vi "InitConfig.vi"() -> ()   [LabVIEW 2014]
uses:
  QMH Fundamentals - Message Cluster.ctl
panel:
  in  "返回2":bool
  in  "标准测试":bool
  in  "自定义测试":bool
  in  "返回":bool
  in  "自动测试":bool
  in  "单次测试":bool
  in  "自定义测试":bool
  in  "常温拷机":bool
  in  "高温老练":bool
  in  "温循":bool
  in  "退出":bool
  in  "手动测试":bool
  in  "全自动测试":bool
  # "请选择测试类型"
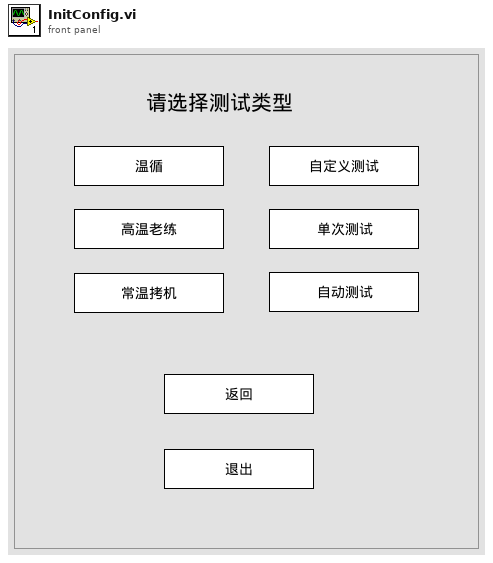
[diagram p1: front panel]
types:
  T1 = typedef "QMH Fundamentals - Message Cluster.ctl" = cluster{"消息":string, "消息数据":variant}
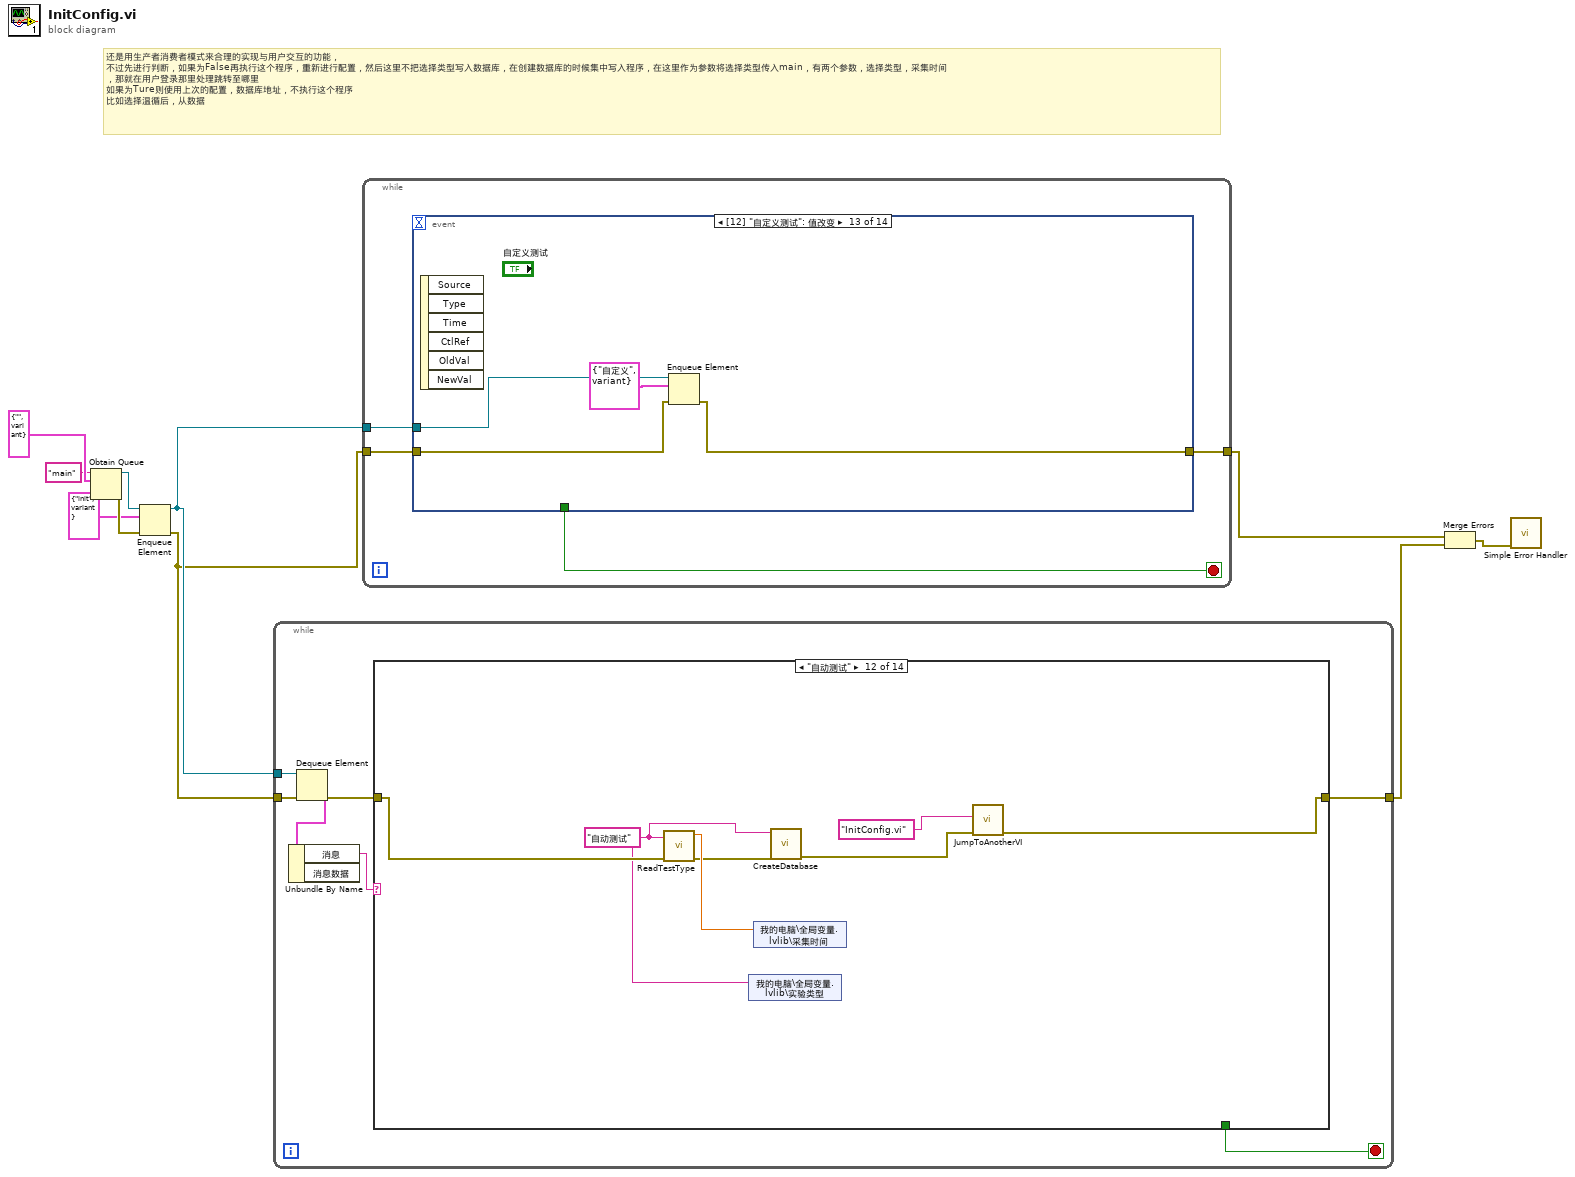
[diagram p0: block diagram]
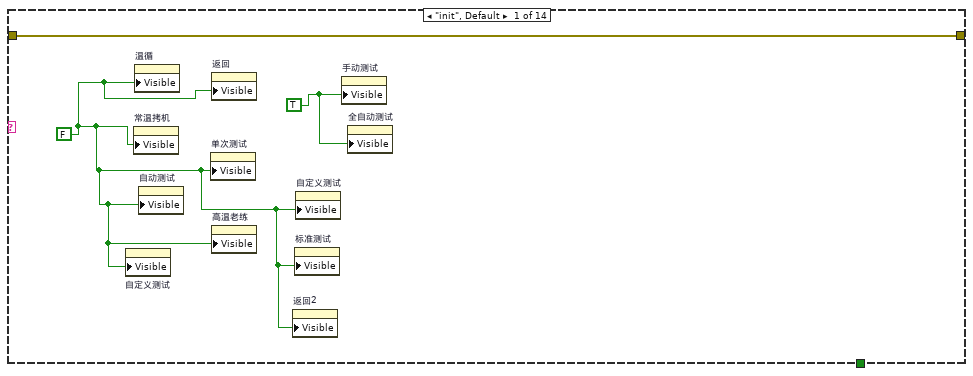
[diagram p2: hidden frame]
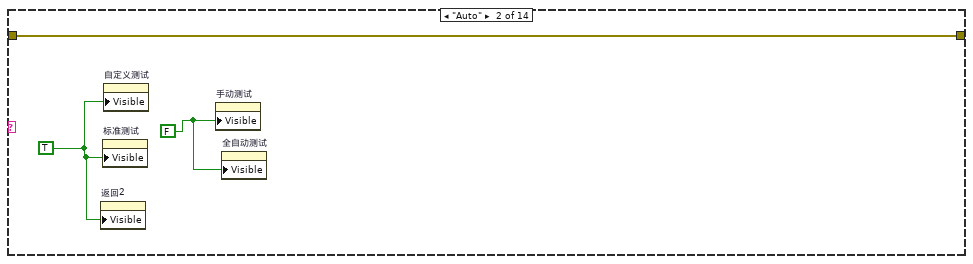
[diagram p3: hidden frame]
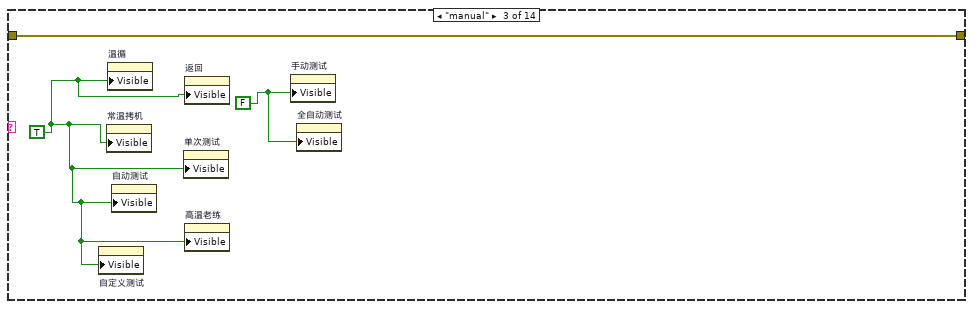
[diagram p4: hidden frame]
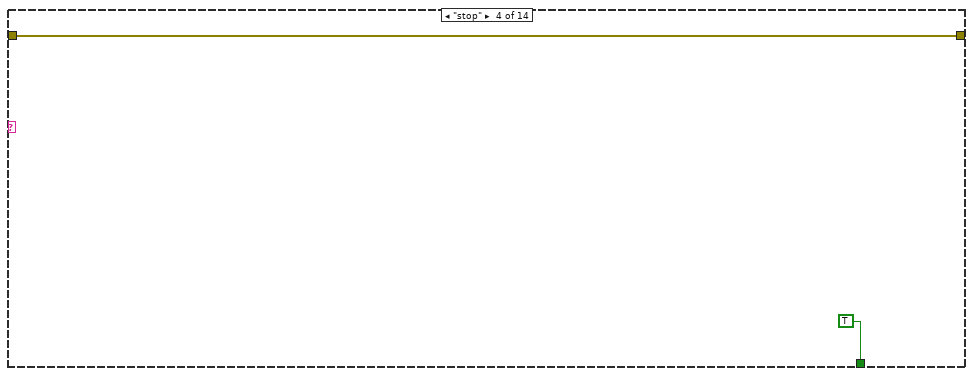
[diagram p5: hidden frame]
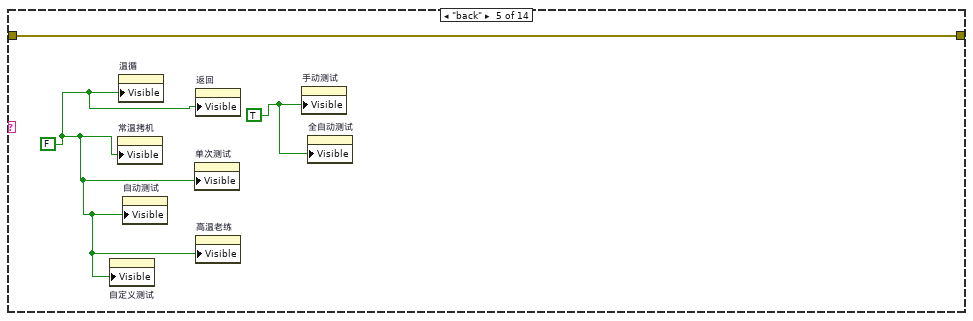
[diagram p6: hidden frame]
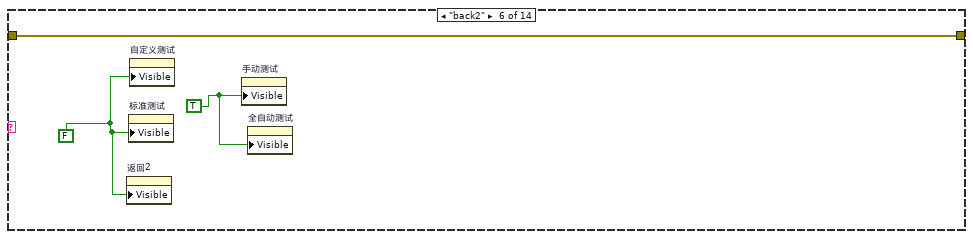
[diagram p7: hidden frame]
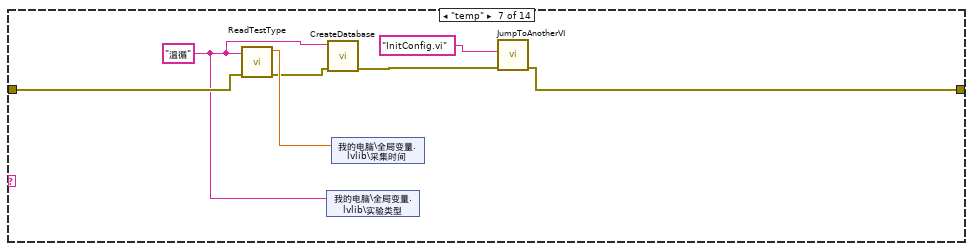
[diagram p8: hidden frame]
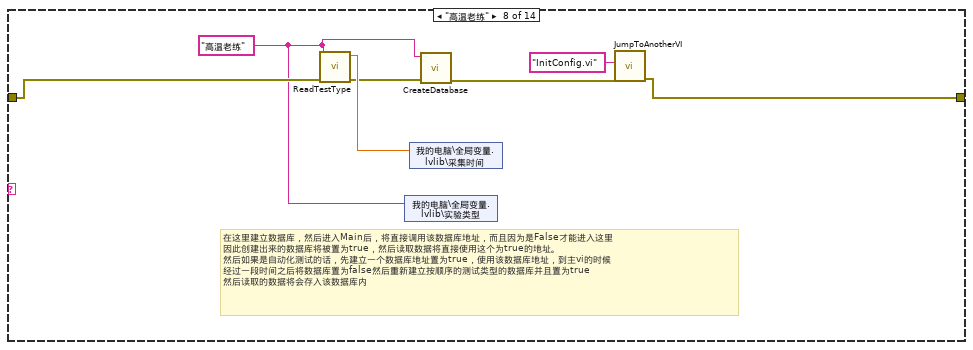
[diagram p9: hidden frame]
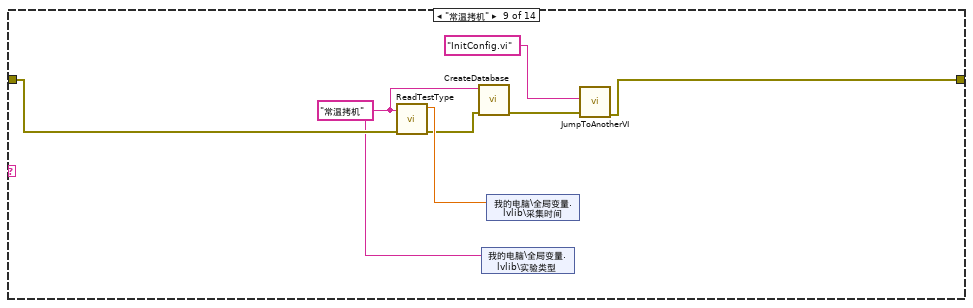
[diagram p10: hidden frame]
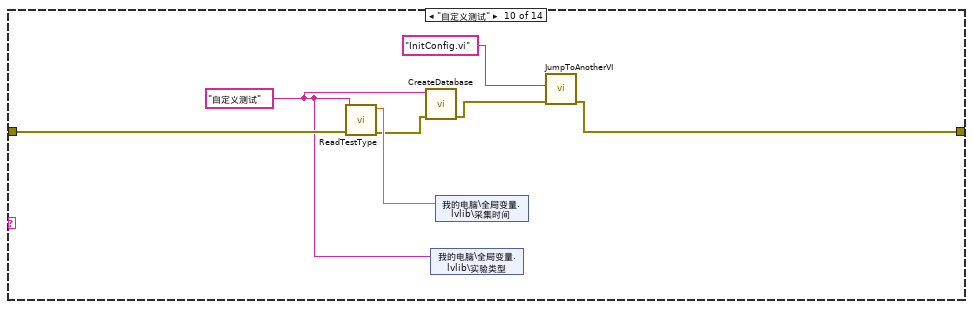
[diagram p11: hidden frame]
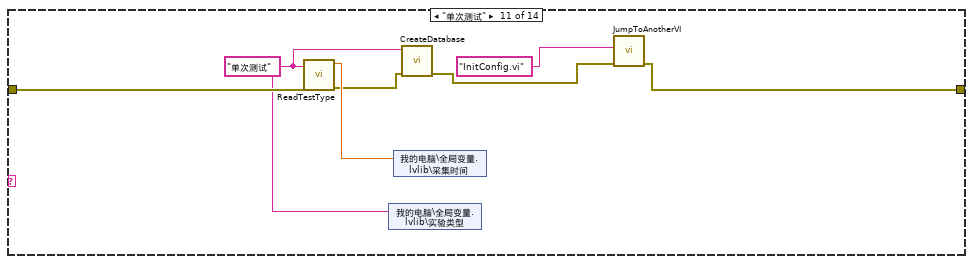
[diagram p12: hidden frame]
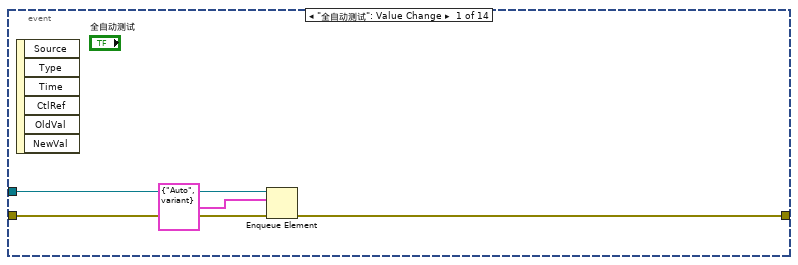
[diagram p15: hidden frame]
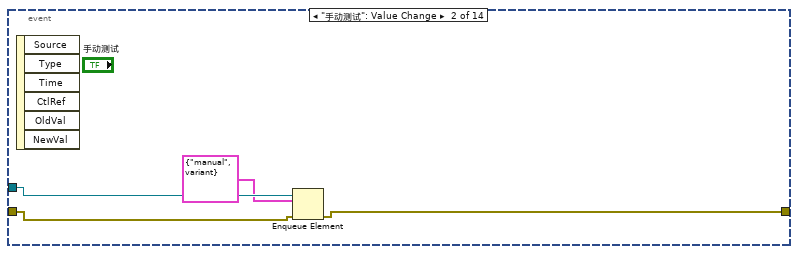
[diagram p16: hidden frame]
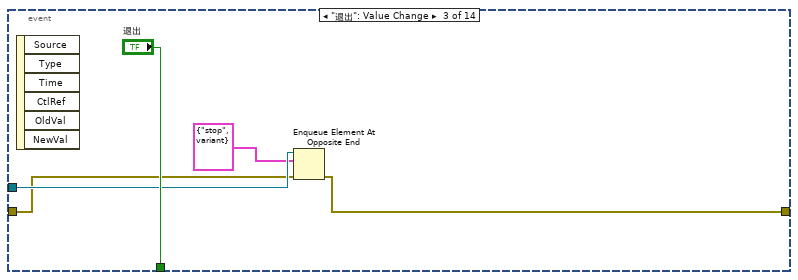
[diagram p17: hidden frame]
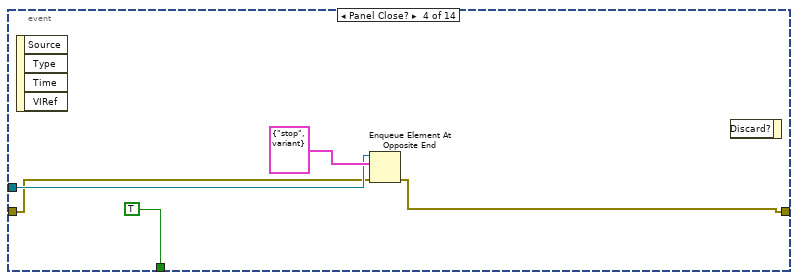
[diagram p18: hidden frame]
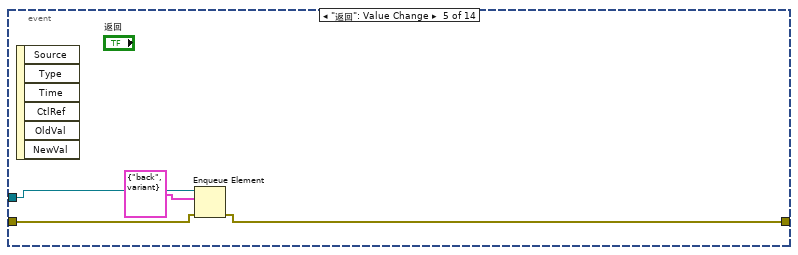
[diagram p19: hidden frame]
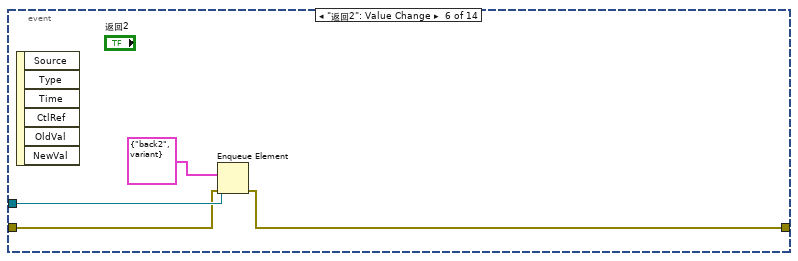
[diagram p20: hidden frame]
diagram:
  # "还是用生产者消费者模式来合理的实现与用户交互的功能，\n不过先进行判断，如果为False再执行这个程序，重新进行配置，然后这里不把选择类型写入数据库，在创建数据库的时候集中写入程序，在这里作为参数将选择类型传入main，有两个参数，选择类型，采集时间\n，那就在用户登录那里处理跳转至哪里\n如果为Ture则使用上次的配置，数据库地址，不执行这个程序\n比如选择温循后，从数据"
  n1 = Obtain Queue(name (unnamed)="main" ("名称（未命名）"), element data type=T1 {"消息"="", "消息数据"=variant} ("消息簇")) -> (queue out=w8:refnum<queue>, error out=w7:errorcluster)  [unwired: 3 in, 1 out]
  n2 = Enqueue Element(queue=w8, element=T1 {"消息"="init", "消息数据"=variant} ("元素"), error in (no error)=w7) -> (queue out=w5:refnum<queue>, error out=w4:errorcluster)  [unwired: 1 in, 1 out]
  n3 = while {
    tunnel: w5 -> [w17]
    tunnel: w4 -> [w16]
    tunnel: [w12] -> w2
    stop <- w11 stop-if-true
    n4 = Dequeue Element(queue=w17, error in (no error)=w16) -> (element=w15:T1, error out=w13:errorcluster)  [unwired: 1 in, 2 out]
    n5 = Unbundle By Name(w15) -> ("消息"=w14:string)  [unwired: 1 out]
    n6 = case shown="\"自动测试\"" w14 {
      tunnel: w13 -> [w20 w23 w26 w28 w29 w32 w41 w47 w54 w61 w68 w75 w77 w78]
      tunnel: [w20 w23 w26 w28 w29 w32 w39 w46 w53 w60 w67 w74 w77 w78] -> w12
      tunnel: [_ _ _ TRUE _ _ _ _ _ _ _ _ _ _] -> w11
      frame "init", Default {
        w19 = TRUE
        w18 = FALSE
        n7 = property on="自定义测试" class="Bool"("Visible"=w18) -> ()  [unwired: 2 in, 2 out]
        n8 = property on="常温拷机" class="Bool"("Visible"=w18) -> ()  [unwired: 2 in, 2 out]
        n9 = property on="温循" class="Bool"("Visible"=w18) -> ()  [unwired: 2 in, 2 out]
        n10 = property on="自动测试" class="Bool"("Visible"=w18) -> ()  [unwired: 2 in, 2 out]
        n11 = property on="单次测试" class="Bool"("Visible"=w18) -> ()  [unwired: 2 in, 2 out]
        n12 = property on="返回" class="Bool"("Visible"=w18) -> ()  [unwired: 2 in, 2 out]
        n13 = property on="高温老练" class="Bool"("Visible"=w18) -> ()  [unwired: 2 in, 2 out]
        n14 = property on="返回2" class="Bool"("Visible"=w18) -> ()  [unwired: 2 in, 2 out]
        n15 = property on="标准测试" class="Bool"("Visible"=w18) -> ()  [unwired: 2 in, 2 out]
        n16 = property on="自定义测试" class="Bool"("Visible"=w18) -> ()  [unwired: 2 in, 2 out]
        n17 = property on="手动测试" class="Bool"("Visible"=w19) -> ()  [unwired: 2 in, 2 out]
        n18 = property on="全自动测试" class="Bool"("Visible"=w19) -> ()  [unwired: 2 in, 2 out]
      }
      frame "Auto" {
        w21 = FALSE
        w22 = TRUE
        n19 = property on="返回2" class="Bool"("Visible"=w22) -> ()  [unwired: 2 in, 2 out]
        n20 = property on="标准测试" class="Bool"("Visible"=w22) -> ()  [unwired: 2 in, 2 out]
        n21 = property on="自定义测试" class="Bool"("Visible"=w22) -> ()  [unwired: 2 in, 2 out]
        n22 = property on="手动测试" class="Bool"("Visible"=w21) -> ()  [unwired: 2 in, 2 out]
        n23 = property on="全自动测试" class="Bool"("Visible"=w21) -> ()  [unwired: 2 in, 2 out]
      }
      frame "manual" {
        w25 = FALSE
        w24 = TRUE
        n24 = property on="自定义测试" class="Bool"("Visible"=w24) -> ()  [unwired: 2 in, 2 out]
        n25 = property on="常温拷机" class="Bool"("Visible"=w24) -> ()  [unwired: 2 in, 2 out]
        n26 = property on="温循" class="Bool"("Visible"=w24) -> ()  [unwired: 2 in, 2 out]
        n27 = property on="自动测试" class="Bool"("Visible"=w24) -> ()  [unwired: 2 in, 2 out]
        n28 = property on="单次测试" class="Bool"("Visible"=w24) -> ()  [unwired: 2 in, 2 out]
        n29 = property on="返回" class="Bool"("Visible"=w24) -> ()  [unwired: 2 in, 2 out]
        n30 = property on="高温老练" class="Bool"("Visible"=w24) -> ()  [unwired: 2 in, 2 out]
        n31 = property on="手动测试" class="Bool"("Visible"=w25) -> ()  [unwired: 2 in, 2 out]
        n32 = property on="全自动测试" class="Bool"("Visible"=w25) -> ()  [unwired: 2 in, 2 out]
      }
      frame "stop" {
      }
      frame "back" {
        w31 = TRUE
        w30 = FALSE
        n33 = property on="自定义测试" class="Bool"("Visible"=w30) -> ()  [unwired: 2 in, 2 out]
        n34 = property on="常温拷机" class="Bool"("Visible"=w30) -> ()  [unwired: 2 in, 2 out]
        n35 = property on="温循" class="Bool"("Visible"=w30) -> ()  [unwired: 2 in, 2 out]
        n36 = property on="自动测试" class="Bool"("Visible"=w30) -> ()  [unwired: 2 in, 2 out]
        n37 = property on="单次测试" class="Bool"("Visible"=w30) -> ()  [unwired: 2 in, 2 out]
        n38 = property on="返回" class="Bool"("Visible"=w30) -> ()  [unwired: 2 in, 2 out]
        n39 = property on="高温老练" class="Bool"("Visible"=w30) -> ()  [unwired: 2 in, 2 out]
        n40 = property on="手动测试" class="Bool"("Visible"=w31) -> ()  [unwired: 2 in, 2 out]
        n41 = property on="全自动测试" class="Bool"("Visible"=w31) -> ()  [unwired: 2 in, 2 out]
      }
      frame "back2" {
        w33 = TRUE
        w34 = FALSE
        n42 = property on="返回2" class="Bool"("Visible"=w34) -> ()  [unwired: 2 in, 2 out]
        n43 = property on="标准测试" class="Bool"("Visible"=w34) -> ()  [unwired: 2 in, 2 out]
        n44 = property on="自定义测试" class="Bool"("Visible"=w34) -> ()  [unwired: 2 in, 2 out]
        n45 = property on="手动测试" class="Bool"("Visible"=w33) -> ()  [unwired: 2 in, 2 out]
        n46 = property on="全自动测试" class="Bool"("Visible"=w33) -> ()  [unwired: 2 in, 2 out]
      }
      frame "temp" {
        w36 = "温循"
        n47 = call "ReadTestType.vi"("error in (no error)"=w41, "列名"=w36) -> ("error out"=w37:errorcluster, "输出 1"=w40:dbl)  [unwired: 8 in]
        n48 = shared-variable "我的电脑\\全局变量.lvlib\\实验类型"(w36) -> ()  [unwired: 1 in, 1 out]
        n49 = call "CreateDatabase.vi"("错误输入（无错误）"=w37, "测试类型"=w36) -> ("error out"=w35:errorcluster)  [unwired: 8 in, 1 out]
        n50 = shared-variable "我的电脑\\全局变量.lvlib\\采集时间"(w40) -> ()  [unwired: 1 in, 1 out]
        n51 = call "JumpToAnotherVI.vi"("错误输入（无错误）"=w35, "要关闭的VI"="InitConfig.vi") -> ("错误输出"=w39:errorcluster)  [unwired: 9 in]
      }
      frame "高温老练" {
        w42 = "高温老练"
        # "在这里建立数据库，然后进入Main后，将直接调用该数据库地址，而且因为是False才能进入这里\n因此创建出来的数据库将被置为true，然后读取数据将直接使用这个为true的地址。\n然后如果是自动化测试的话，先建立一个数据库地址置为true，使用该数据库地址，到主vi的时候\n经过一段时间之后将数据库置为false然后重新建立按顺序的测试类型的数据库并且置为true\n然后读取的数据将会存入该数据库内"
        n52 = call "ReadTestType.vi"("error in (no error)"=w47, "列名"=w42) -> ("error out"=w44:errorcluster, "输出 1"=w48:dbl)  [unwired: 8 in]
        n53 = shared-variable "我的电脑\\全局变量.lvlib\\实验类型"(w42) -> ()  [unwired: 1 in, 1 out]
        n54 = shared-variable "我的电脑\\全局变量.lvlib\\采集时间"(w48) -> ()  [unwired: 1 in, 1 out]
        n55 = call "CreateDatabase.vi"("错误输入（无错误）"=w44, "测试类型"=w42) -> ("error out"=w43:errorcluster)  [unwired: 8 in, 1 out]
        n56 = call "JumpToAnotherVI.vi"("错误输入（无错误）"=w43, "要关闭的VI"="InitConfig.vi") -> ("错误输出"=w46:errorcluster)  [unwired: 9 in]
      }
      frame "常温拷机" {
        w49 = "常温拷机"
        n57 = call "ReadTestType.vi"("error in (no error)"=w54, "列名"=w49) -> ("error out"=w51:errorcluster, "输出 1"=w55:dbl)  [unwired: 8 in]
        n58 = call "CreateDatabase.vi"("错误输入（无错误）"=w51, "测试类型"=w49) -> ("error out"=w50:errorcluster)  [unwired: 8 in, 1 out]
        n59 = shared-variable "我的电脑\\全局变量.lvlib\\实验类型"(w49) -> ()  [unwired: 1 in, 1 out]
        n60 = shared-variable "我的电脑\\全局变量.lvlib\\采集时间"(w55) -> ()  [unwired: 1 in, 1 out]
        n61 = call "JumpToAnotherVI.vi"("错误输入（无错误）"=w50, "要关闭的VI"="InitConfig.vi") -> ("错误输出"=w53:errorcluster)  [unwired: 9 in]
      }
      frame "自定义测试" {
        w56 = "自定义测试"
        n62 = call "ReadTestType.vi"("error in (no error)"=w61, "列名"=w56) -> ("error out"=w58:errorcluster, "输出 1"=w62:dbl)  [unwired: 8 in]
        n63 = call "CreateDatabase.vi"("错误输入（无错误）"=w58, "测试类型"=w56) -> ("error out"=w57:errorcluster)  [unwired: 8 in, 1 out]
        n64 = shared-variable "我的电脑\\全局变量.lvlib\\实验类型"(w56) -> ()  [unwired: 1 in, 1 out]
        n65 = shared-variable "我的电脑\\全局变量.lvlib\\采集时间"(w62) -> ()  [unwired: 1 in, 1 out]
        n66 = call "JumpToAnotherVI.vi"("错误输入（无错误）"=w57, "要关闭的VI"="InitConfig.vi") -> ("错误输出"=w60:errorcluster)  [unwired: 9 in]
      }
      frame "单次测试" {
        w63 = "单次测试"
        n67 = call "ReadTestType.vi"("error in (no error)"=w68, "列名"=w63) -> ("error out"=w65:errorcluster, "输出 1"=w69:dbl)  [unwired: 8 in]
        n68 = shared-variable "我的电脑\\全局变量.lvlib\\实验类型"(w63) -> ()  [unwired: 1 in, 1 out]
        n69 = shared-variable "我的电脑\\全局变量.lvlib\\采集时间"(w69) -> ()  [unwired: 1 in, 1 out]
        n70 = call "CreateDatabase.vi"("错误输入（无错误）"=w65, "测试类型"=w63) -> ("error out"=w64:errorcluster)  [unwired: 8 in, 1 out]
        n71 = call "JumpToAnotherVI.vi"("错误输入（无错误）"=w64, "要关闭的VI"="InitConfig.vi") -> ("错误输出"=w67:errorcluster)  [unwired: 9 in]
      }
      frame "自动测试" {
        w70 = "自动测试"
        n72 = call "ReadTestType.vi"("error in (no error)"=w75, "列名"=w70) -> ("error out"=w72:errorcluster, "输出 1"=w76:dbl)  [unwired: 8 in]
        n73 = shared-variable "我的电脑\\全局变量.lvlib\\实验类型"(w70) -> ()  [unwired: 1 in, 1 out]
        n74 = shared-variable "我的电脑\\全局变量.lvlib\\采集时间"(w76) -> ()  [unwired: 1 in, 1 out]
        n75 = call "CreateDatabase.vi"("错误输入（无错误）"=w72, "测试类型"=w70) -> ("error out"=w71:errorcluster)  [unwired: 8 in, 1 out]
        n76 = call "JumpToAnotherVI.vi"("错误输入（无错误）"=w71, "要关闭的VI"="InitConfig.vi") -> ("错误输出"=w74:errorcluster)  [unwired: 9 in]
      }
      frame "自定义" {
      }
      frame "标准测试" {
      }
    }
  }
  n77 = while {
    tunnel: w5 -> [w81]
    tunnel: w4 -> [w80]
    tunnel: [w79] -> w3
    stop <- w82 stop-if-true
    n78 = event shown="[12] \"自定义测试\": 值改变" {
      selector: _ -> [_ _ _ _ _ _ _ _ _ _ _ _ _ _]
      dyn-events: _ -> [_ _ _ _ _ _ _ _ _ _ _ _ _ _]
      timeout: _ -> [_ _ _ _ _ _ _ _ _ _ _ _ _ _]
      tunnel: [_ _ "退出" TRUE _ _ _ _ _ _ _ _ _ _] -> w82
      tunnel: w81 -> [w86 w90 w94 w98 w104 w108 w112 w115 w119 w123 w127 w131 w135 w139]
      tunnel: w80 -> [w85 w89 w93 w97 w103 w107 w111 w114 w118 w122 w126 w130 w134 w138]
      tunnel: [w83 w88 w91 w96 w102 w105 w110 w113 w117 w121 w125 w129 w133 w137] -> w79
      event "全自动测试": Value Change {
        n79 = event-data() -> ()  [unwired: 1 in, 6 out]
        n80 = Enqueue Element(queue=w86, element=T1 {"消息"="Auto", "消息数据"=variant} ("元素"), error in (no error)=w85) -> (error out=w83:errorcluster)  [unwired: 1 in, 2 out]
      }
      event "手动测试": Value Change {
        n81 = event-data() -> ()  [unwired: 1 in, 6 out]
        n82 = Enqueue Element(queue=w90, element=T1 {"消息"="manual", "消息数据"=variant} ("元素"), error in (no error)=w89) -> (error out=w88:errorcluster)  [unwired: 1 in, 2 out]
      }
      event "退出": Value Change {
        n83 = event-data() -> ()  [unwired: 1 in, 6 out]
        n84 = Enqueue Element At Opposite End(queue=w94, element=T1 {"消息"="stop", "消息数据"=variant} ("元素"), error in (no error)=w93) -> (error out=w91:errorcluster)  [unwired: 1 in, 2 out]
      }
      event Panel Close? {
        n85 = event-data() -> ()  [unwired: 1 in, 4 out]
        n86 = Enqueue Element At Opposite End(queue=w98, element=T1 {"消息"="stop", "消息数据"=variant} ("元素"), error in (no error)=w97) -> (error out=w96:errorcluster)  [unwired: 1 in, 2 out]
        n87 = event-data() -> ()  [unwired: 2 in, 1 out]
      }
      event "返回": Value Change {
        n88 = event-data() -> ()  [unwired: 1 in, 6 out]
        n89 = Enqueue Element(queue=w104, element=T1 {"消息"="back", "消息数据"=variant} ("元素"), error in (no error)=w103) -> (error out=w102:errorcluster)  [unwired: 1 in, 2 out]
      }
      event "返回2": Value Change {
        n90 = event-data() -> ()  [unwired: 1 in, 6 out]
        n91 = Enqueue Element(queue=w108, element=T1 {"消息"="back2", "消息数据"=variant} ("元素"), error in (no error)=w107) -> (error out=w105:errorcluster)  [unwired: 1 in, 2 out]
      }
      event "温循": Value Change {
        n92 = event-data() -> ()  [unwired: 1 in, 6 out]
        n93 = Enqueue Element(queue=w112, element=T1 {"消息"="temp", "消息数据"=variant} ("元素"), error in (no error)=w111) -> (error out=w110:errorcluster)  [unwired: 1 in, 2 out]
      }
      event "高温老练": Value Change {
        n94 = event-data() -> ()  [unwired: 1 in, 6 out]
        n95 = Enqueue Element(queue=w115, element=T1 {"消息"="高温老练", "消息数据"=variant} ("元素"), error in (no error)=w114) -> (error out=w113:errorcluster)  [unwired: 1 in, 2 out]
      }
      event "常温拷机": Value Change {
        n96 = event-data() -> ()  [unwired: 1 in, 6 out]
        n97 = Enqueue Element(queue=w119, element=T1 {"消息"="常温拷机", "消息数据"=variant} ("元素"), error in (no error)=w118) -> (error out=w117:errorcluster)  [unwired: 1 in, 2 out]
      }
      event "自定义测试": Value Change {
        n98 = event-data() -> ()  [unwired: 1 in, 6 out]
        n99 = Enqueue Element(queue=w123, element=T1 {"消息"="自定义测试", "消息数据"=variant} ("元素"), error in (no error)=w122) -> (error out=w121:errorcluster)  [unwired: 1 in, 2 out]
      }
      event "单次测试": Value Change {
        n100 = event-data() -> ()  [unwired: 1 in, 6 out]
        n101 = Enqueue Element(queue=w127, element=T1 {"消息"="单次测试", "消息数据"=variant} ("元素"), error in (no error)=w126) -> (error out=w125:errorcluster)  [unwired: 1 in, 2 out]
      }
      event "自动测试": Value Change {
        n102 = event-data() -> ()  [unwired: 1 in, 6 out]
        n103 = Enqueue Element(queue=w131, element=T1 {"消息"="自动测试", "消息数据"=variant} ("元素"), error in (no error)=w130) -> (error out=w129:errorcluster)  [unwired: 1 in, 2 out]
      }
      event "自定义测试": Value Change {
        n104 = event-data() -> ()  [unwired: 1 in, 6 out]
        n105 = Enqueue Element(queue=w135, element=T1 {"消息"="自定义", "消息数据"=variant} ("元素"), error in (no error)=w134) -> (error out=w133:errorcluster)  [unwired: 1 in, 2 out]
      }
      event "标准测试": Value Change {
        n106 = event-data() -> ()  [unwired: 1 in, 6 out]
        n107 = Enqueue Element(queue=w139, element=T1 {"消息"="标准测试", "消息数据"=variant} ("元素"), error in (no error)=w138) -> (error out=w137:errorcluster)  [unwired: 1 in, 2 out]
      }
    }
  }
  n108 = Merge Errors(w3, w2) -> (w1:errorcluster)
  n109 = call <vilib>:"Simple Error Handler.vi"("error in (no error)"=w1) -> ()  [unwired: 4 in, 5 out]
